vi "sim_interpolate_iCorr.vi"(7 "point in":dbl[](array[numeric]), 8 "nPts in":dbl, 9 "sim-pdy":dbl[](array[numeric]), 10 "sim-pdx":dbl[](array[numeric]), 11 "sim-iCorr":dbl[](array[numeric])) -> (0 "nPts out":dbl, 2 "iCorr out":dbl, 5 "measured-point out":dbl[](array[numeric]))   [LabVIEW 2024]
uses:
  <vilib>/gmath/interp.llb/Interpolate 2D Scattered (1D).vi
  <vilib>/gmath/NI_AAL_Interpolation.lvlib
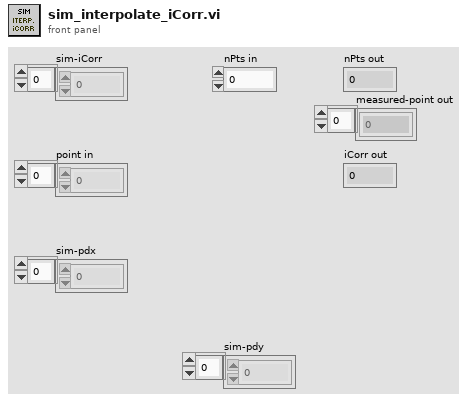
[diagram p1: front panel]
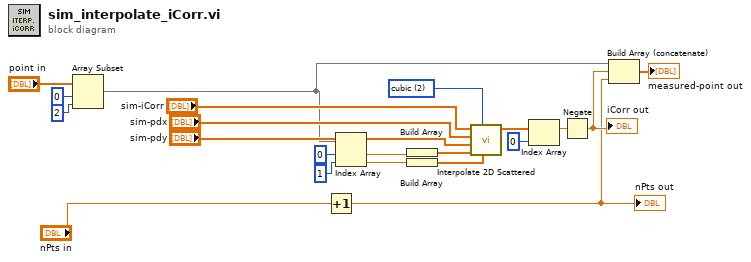
[diagram p0: block diagram]
diagram:
  w8 = 2 items=["nearest", "linear", "cubic", "biharmonic spline "] ("method")
  n1 = Array Subset(array="point in", index=0, length=2) -> (w4:dbl[])
  n2 = Increment(x="nPts in") -> (x+1=w2:dbl)
  "nPts out" <- w2
  n3 = Index Array(array=w4, index #1=0 ("index"), index #2=1 ("index")) -> (element #1=w14:dbl, element #2=w16:dbl)
  n4 = Build Array(w14) -> (w15:dbl[])
  n5 = Build Array(w16) -> (w17:dbl[])
  n6 = call-poly <vilib>:"Interpolate 2D Scattered.vi"("Yi"=w17, "method"=w8, "Xi"=w15, "Y"="sim-pdy", "X"="sim-pdx", "Z"="sim-iCorr") -> ("Zi"=w18:dbl[])  [unwired: 4 in, 1 out]
  n7 = Index Array(array=w18, index=0) -> (element=w21:dbl)
  n8 = Negate(x=w21) -> (-x=w3:dbl)
  "iCorr out" <- w3
  n9 = Build Array (concatenate)(w4, w3, w2) -> (→"measured-point out":dbl[])
